vi "Actor Core.vi"(8 "error in":errorcluster, 11 "Actor in":refnum<class "Actor.lvclass">) -> (0 "error out":errorcluster, 3 "Actor out":refnum<class "Actor.lvclass">)   [LabVIEW 2020, in "Actor Framework.lvlib" / "Actor.lvclass"]
doc: "<p>(<strong>Filename</strong>: <span class=\"dnl\">Actor Framework.lvlib:Actor.lvclass:Actor Core.vi</span>)</p>\n<p>Receives messages to the actor, reacts to them, and initiates any error handling that may shut the actor down.</p>\n<p>Descendant classes may override this VI to append parallel tasks for the actor to complete while it handles messages. Overrides use the <a href=\"nihelplauncher://docs/csh?context=lvcore_glang_udclass\">Call Parent Class Method</a> node.</p>"
uses:
  Actor.lvclass
  Actor.lvclass/Actor.ctl
  Message Priority Queue/Message Priority Queue.lvclass
  Actor Framework.lvlib
  tracing/Support/Registration Mode.ctl
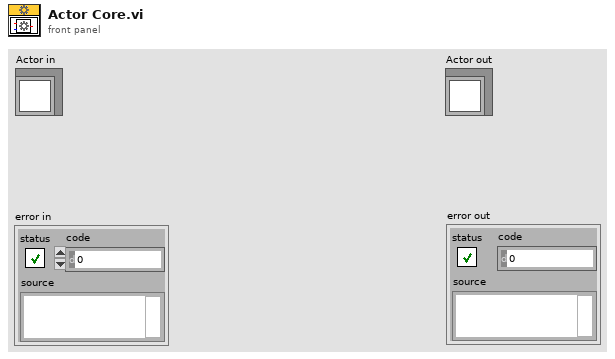
[diagram p1: front panel]
types:
  T1 = typedef "Actor Framework.lvlib/Registration Mode.ctl" = enum16{"Register Actor", "Get ID", "Get Enqueuer", "Deregister Actor", "Get Update Event", "Get All Actors", "Set Actor Core Name"}
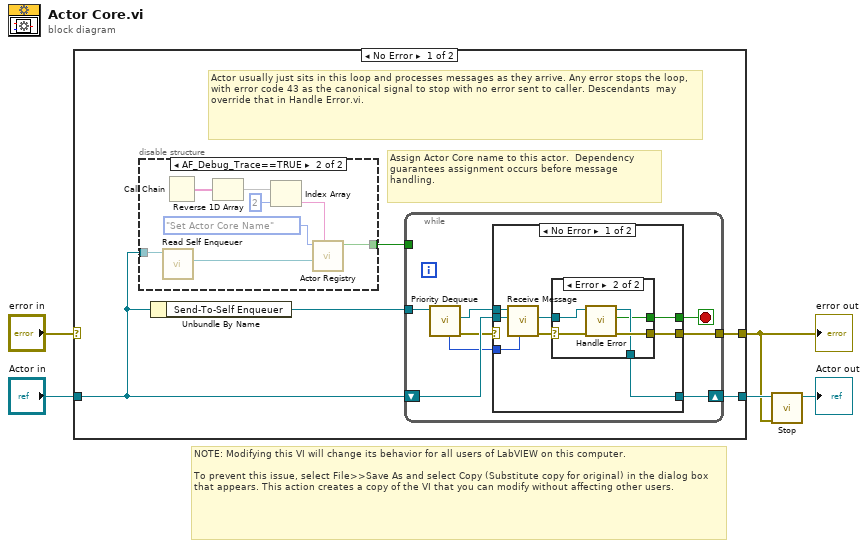
[diagram p0: block diagram]
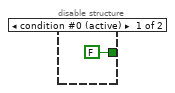
[diagram p2: hidden frame]
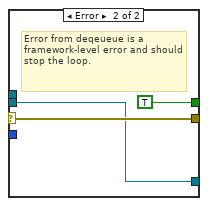
[diagram p4: hidden frame]
diagram:
  # "NOTE: Modifying this VI will change its behavior for all users of LabVIEW on this computer.\n\nTo prevent this issue, select File>>Save As and select Copy (Substitute copy for original) in the dialog box that appears. This action creates a copy of the VI that you can modify without affecting other users."
  n1 = case shown="No Error" "error in" {
    selector: "error in" -> [_ w47]
    tunnel: [w8 w47] -> w1
    tunnel: "Actor in" -> [w7 w46]
    tunnel: [w9 w46] -> w3
    frame No Error {
      # "Assign Actor Core name to this actor.  Dependency guarantees assignment occurs before message handling."
      # "Actor usually just sits in this loop and processes messages as they arrive. Any error stops the loop, with error code 43 as the canonical signal to stop with no error sent to caller. Descendants  may override that in Handle Error.vi."
      n2 = disable-structure shown="AF_Debug_Trace==TRUE" {
        disable-tunnel: w7 -> [_ w19]
        disable-tunnel: [FALSE ("Found") w12] -> w6
        frame condition #0 (active) {
        }
        frame condition #1 {
          n3 = call "Read Self Enqueuer.vi"("Actor"=w19) -> ("Self Enqueuer"=w13:refnum<class "Message Enqueuer.lvclass">)  [unwired: 10 in]
          n4 = Call Chain() -> (call chain=w16:string[])
          n5 = Reverse 1D Array(array=w16) -> (reversed array=w17:string[])
          n6 = Index Array(array=w17, index=2) -> (element=w18:string)
          n7 = call "Actor Registry.vi"("Actor Core Name"=w18, "Actor Enqueuer"=w13, "Action"=Registration_Mode."Set Actor Core Name") -> ("Found"=w12:bool)  [unwired: 4 in, 4 out]
        }
      }
      n8 = Unbundle By Name(w7) -> ("Send-To-Self Enqueuer"=w10:refnum<class "Message Priority Queue.lvclass">)
      n9 = while {
        tunnel: w10 -> [w25]
        shift-right: [w22] -> w9
        shift-left: w7 -> [w27]
        tunnel: [w20] -> w8
        tunnel: w6 -> [_]
        stop <- w21 stop-if-true
        n10 = call "Priority Dequeue.vi"("Priority Queue in"=w25) -> ("error out"=w23:errorcluster, "element"=w26:refnum<class "Message.lvclass">, "priority"=w24:i32)  [unwired: 6 in, 2 out]
        n11 = case shown="No Error" w23 {
          selector: w23 -> [_ w45]
          tunnel: w27 -> [w35 w44]
          tunnel: w26 -> [w34 _]
          tunnel: [w29 w45] -> w20
          tunnel: [w30 TRUE] -> w21
          tunnel: w24 -> [w33 _]
          tunnel: [w28 w44] -> w22
          frame No Error {
            n12 = call-dynamic "Receive Message.vi"("priority"=w33, "Actor in"=w35, "Message in"=w34) -> ("error out"=w32:errorcluster, "Actor out"=w31:refnum<class "Actor.lvclass">)  [unwired: 7 in]
            n13 = case shown="Error" w32 {
              selector: w32 -> [w36 w39]
              tunnel: [w36 w42] -> w29
              tunnel: w31 -> [w37 w41]
              tunnel: [w37 w40] -> w28
              tunnel: [_ w38] -> w30
              frame No Error {
              }
              frame Error {
                n14 = call-dynamic "Handle Error.vi"("error in (no error)"=w39, "Actor in"=w41) -> ("error out"=w42:errorcluster, "stop actor?"=w38:bool, "Actor out"=w40:refnum<class "Actor.lvclass">)  [unwired: 7 in]
              }
            }
          }
          frame Error {
            # "Error from deqeueue is a framework-level error and should stop the loop."
          }
        }
      }
    }
    frame Error {
    }
  }
  "error out" <- w1
  n15 = call "Stop.vi"("error in"=w1, "Actor in"=w3) -> ("Actor out"=→"Actor out":refnum<class "Actor.lvclass">)  [unwired: 9 in]
